vi "LoadLastLogFileInContext.vi"(8 "error in (no error)":errorcluster, 11 "AppContextIn":T1) -> (0 "error out":errorcluster, 3 "AppContextOut":T1)   [LabVIEW 2013, in "ErrorMessage.lvclass"]
uses:
  001 - MAIN/Class/Messages/ErrorMessage/ErrorMessage.lvclass
  MessageHandlerContext.ctl
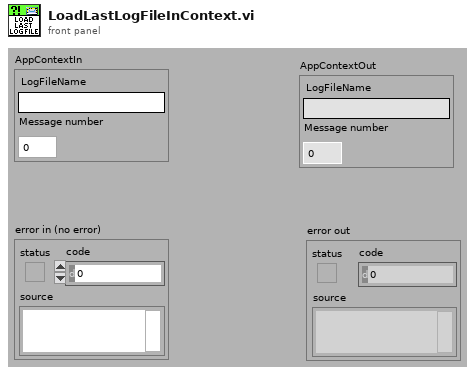
[diagram p1: front panel]
types:
  T1 = typedef "MessageHandlerContext.ctl" = cluster{"LogFileName":string, "Message number":i32}
  T2 = typedef "ErrorMessage.lvclass/LogFileData.ctl" = cluster{"MessageArray":T3[]}
  T3 = typedef "ToMessageHandlerEvent.ctl" = cluster{"date / time":timestamp, "Criticity":T4, "Emitter":string, "Message":string}
  T4 = typedef "enumMessageCriticity.ctl" = enum16{"No error", "Info", "Warning", "Error", "Fatal error"}
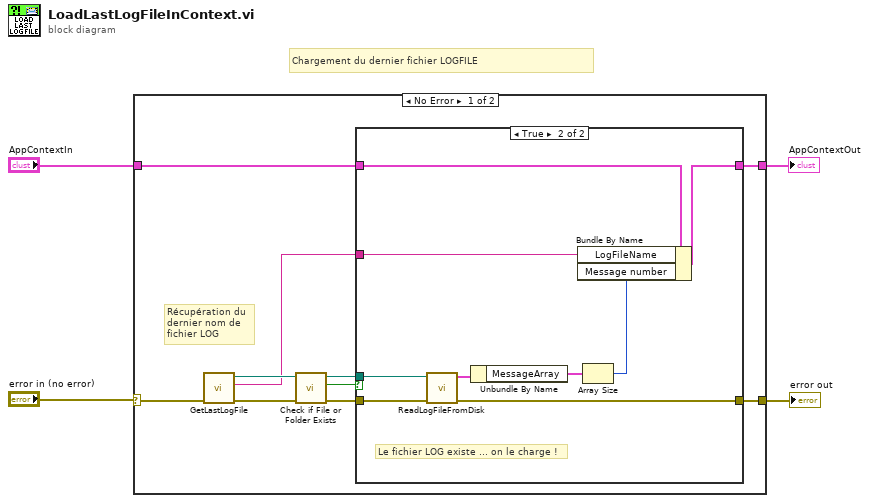
[diagram p0: block diagram]
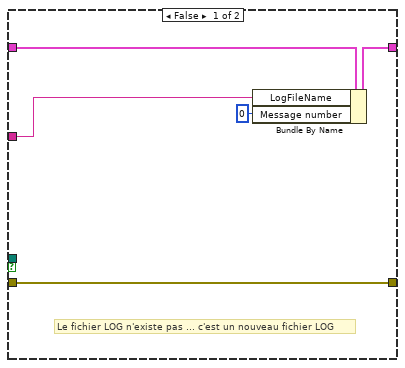
[diagram p2: hidden frame]
diagram:
  # "Chargement du dernier fichier LOGFILE"
  n1 = case shown="No Error" "error in (no error)" {
    selector: "error in (no error)" -> [w14 w30]
    tunnel: [w7 w30] -> w3
    tunnel: "AppContextIn" -> [w9 w29]
    tunnel: [w6 w29] -> w1
    frame No Error {
      # "Récupération du\ndernier nom de \nfichier LOG"
      n2 = call "GetLastLogFile.vi"("error in (no error)"=w14) -> ("error out"=w13:errorcluster, "Last log file name"=w8:string, "Last log file path"=w10:path)  [unwired: 8 in]
      n3 = call <vilib>:"Check if File or Folder Exists.vi"("error in (no error)"=w13, "path"=w10) -> ("error out"=w11:errorcluster, "file or folder exists?"=w12:bool, "dup path"=w5:path)  [unwired: 7 in]
      n4 = case shown="True" w12 {
        tunnel: w11 -> [w17 w28]
        tunnel: w9 -> [w19 w26]
        tunnel: w8 -> [w18 w25]
        tunnel: [w17 w24] -> w7
        tunnel: [w16 w23] -> w6
        tunnel: w5 -> [_ w27]
        frame False {
          # "Le fichier LOG n'existe pas ... c'est un nouveau fichier LOG"
          n5 = Bundle By Name(cluster=w19, "LogFileName"=w18, "Message number"=0) -> (w16:T1)
        }
        frame True {
          # "Le fichier LOG existe ... on le charge !"
          n6 = call "ReadLogFileFromDisk.vi"("error in (no error)"=w28, "Log File path"=w27) -> ("error out"=w24:errorcluster, "Messages"=w22:T2)  [unwired: 8 in]
          n7 = Unbundle By Name(w22) -> ("MessageArray"=w21:T3[])
          n8 = Array Size(array=w21) -> (size(s)=w20:i32)
          n9 = Bundle By Name(cluster=w26, "LogFileName"=w25, "Message number"=w20) -> (w23:T1)
        }
      }
    }
    frame Error {
    }
  }
  "error out" <- w3
  "AppContextOut" <- w1
